vi "matlab_locale.vi"() -> (0 "datetime":string)   [LabVIEW 2019]
panel:
  out "locale datetime":string
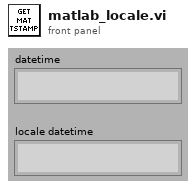
[diagram p1: front panel]
types:
  T1 = typedef "LVDateTimeRec.ctl" = cluster{"fractional second":dbl, "second":i32, "minute":i32, "hour":i32, "day of month":i32, "month":i32, "year":i32, "day of week":i32, "day of year":i32, "DST":i32}
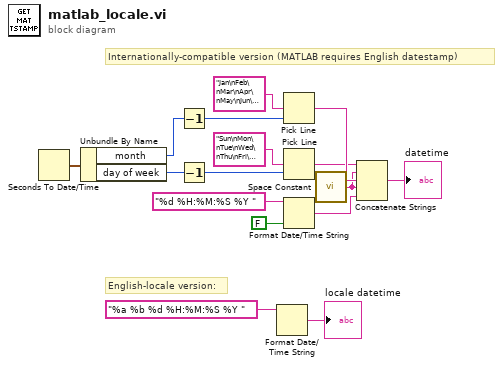
[diagram p0: block diagram]
diagram:
  # "Internationally-compatible version (MATLAB requires English datestamp)"
  # "English-locale version:"
  n1 = Seconds To Date/Time() -> (date time rec=w5:T1)  [unwired: 2 in]
  n2 = Unbundle By Name(w5) -> ("month"=w3:i32, "day of week"=w4:i32)
  n3 = Decrement(x=w3) -> (x-1=w6:i32)
  n4 = Decrement(x=w4) -> (x-1=w1:i32)
  n5 = Format Date/Time String(time format string (%c)="%a %b %d %H:%M:%S %Y ") -> (date/time string=→"locale datetime":string)  [unwired: 2 in]
  n6 = Pick Line(multi-line string="Jan\nFeb\nMar\nApr\nMay\nJun\nJul\nAug\nSep\nOct\nNov\nDec", line index=w6) -> (output string=w13:string)  [unwired: 1 in]
  n7 = Pick Line(multi-line string="Sun\nMon\nTue\nWed\nThu\nFri\nSat", line index=w1) -> (output string=w12:string)  [unwired: 1 in]
  n8 = Format Date/Time String(time format string (%c)="%d %H:%M:%S %Y ", UTC format=FALSE) -> (date/time string=w11:string)  [unwired: 1 in]
  n9 = call <vilib>:"Space Constant.vi"() -> ("String"=w10:string)
  n10 = Concatenate Strings(w12, w10, w13, w10, w11) -> (→"datetime":string)
